vi "Analyze Data.vi"(8 "error in":errorcluster, 11 "tCRD in":refnum<class "Open Path CRD.lvclass">) -> (0 "error out":errorcluster, 3 "tCRD out":refnum<class "Open Path CRD.lvclass">)   [LabVIEW 2015, in "Open Path CRD.lvclass"]
doc: "Analyze Data takes the stored ringdown data (1000 shots per cell) and:\n1) Calculates the ringdown decay constant tau\n2) Averages tau0 data as necessary\n3) Corrects the tau data for Rayleigh scattering\n4) Stores a 1-D array of taus returned on a 1 kHz basis (8k taus) if a jump drive (U:) is connected\n5) Flattens the data into a string and stuffs the string into the <b>data</b> shared variable for display on the UI.\n\nThis VI will not be called if the data is not \"good\" (that is, if an error was thrown in the <B>Get Data</B> routine. If an error is thrown while the data is being retrieved, then the data will not be sent to the UI."
uses:
  Open Path CRD.lvclass
  Reusable/CRDS/Main/CRDS.lvclass
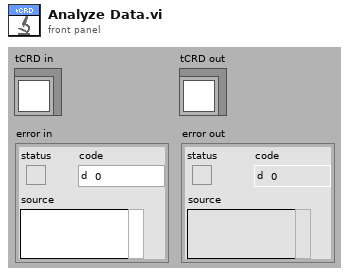
[diagram p1: front panel]
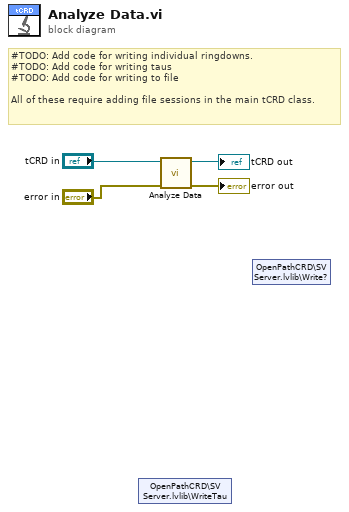
[diagram p0: block diagram]
diagram:
  # "#TODO: Add code for writing individual ringdowns.\n#TODO: Add code for writing taus\n#TODO: Add code for writing to file\n\nAll of these require adding file sessions in the main tCRD class."
  n1 = shared-variable "OpenPathCRD\\SV Server.lvlib\\WriteTau"() -> ()  [unwired: 1 in, 2 out]
  n2 = call-parent "Analyze Data.vi"("error in"="error in", "CRDS in"="tCRD in") -> ("error out"=→"error out":errorcluster, "CRDS out"=→"tCRD out":refnum<class "Open Path CRD.lvclass">)  [unwired: 8 in]
  n3 = shared-variable "OpenPathCRD\\SV Server.lvlib\\Write?"() -> ()  [unwired: 1 in, 2 out]
